vi "Receive.vi"(10 "Msg in":refnum<class "Msg.lvclass">, 11 "Error State in":refnum<class "Error State.lvclass">) -> (2 "Msg out":refnum<class "Msg.lvclass">)   [LabVIEW 2021, in "jettl.lvlib" / "jettl Queue Actor.lvlib" / "Error State.lvclass"]
uses:
  Error State.lvclass
  Actor/Msg/Msg.lvclass
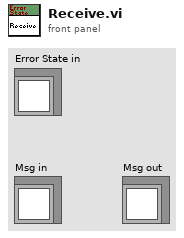
[diagram p1: front panel]
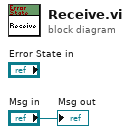
[diagram p0: block diagram]
diagram:
  "Msg out" <- "Msg in"
